vi "Drive Train.vi"(0 "C":dbl format="%#_13g", 1 "D":dbl format="%#_13g", 2 "X":dbl format="%#_13g", 3 "Y":dbl format="%#_13g", 4 "gyro":dbl, 6 "Mode Switch":bool, 7 "Positive 1":bool, 8 "Turning Switch":bool, 9 "Negative 1":bool=TRUE) -> (12 "gyro angle":dbl, 14 "A":dbl, 15 "B":dbl, 16 "R":dbl format="%#_13g")   [LabVIEW 2014]
panel:
  in  "alpha":dbl=1.0 step=0.1
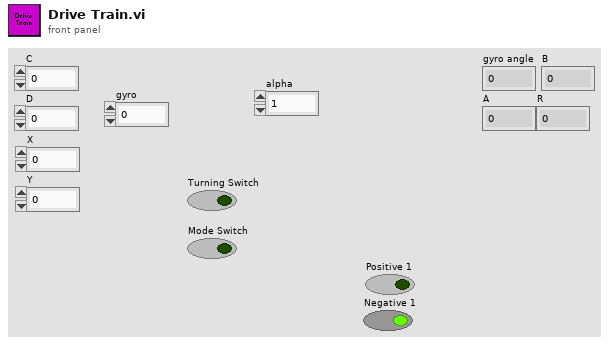
[diagram p1: front panel]
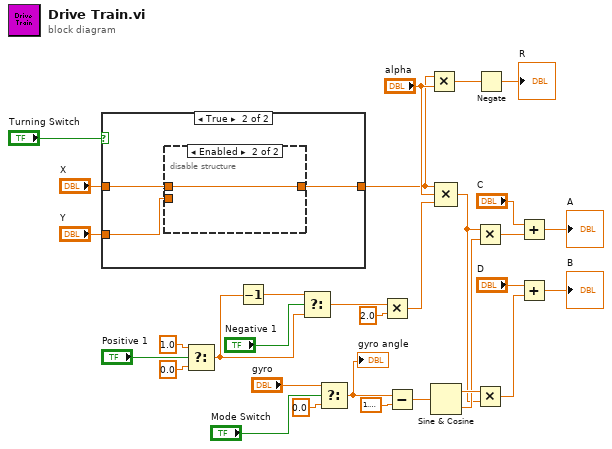
[diagram p0: block diagram]
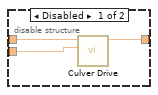
[diagram p3: hidden frame]
diagram:
  n1 = case shown="True" "Turning Switch" {
    tunnel: [w32 w33] -> w6
    tunnel: "X" -> [w32 w34]
    tunnel: "Y" -> [_ w35]
    frame False {
    }
    frame True {
      n2 = disable-structure shown="Enabled" {
        disable-tunnel: w35 -> [w38 _]
        disable-tunnel: w34 -> [w37 w39]
        disable-tunnel: [w36 w39] -> w33
        frame Disabled {
          n3 = call "Culver Drive.vi"("X"=w37, "Y"=w38) -> ("R"=w36:ext)  [unwired: 8 in]
        }
        frame Enabled {
        }
      }
    }
  }
  n4 = Select(t=1.0, s="Positive 1", f=0.0) -> (s? t:f=w15:dbl)
  n5 = Decrement(x=w15) -> (x-1=w14:dbl)
  n6 = Select(t=w14, s="Negative 1", f=w15) -> (s? t:f=w5:dbl)
  n7 = Select(t="gyro", s="Mode Switch", f=0.0 ("t")) -> (s? t:f=w23:dbl)
  "gyro angle" <- w23
  n8 = Multiply(x=w5, y=2.0) -> (x*y=w4:dbl)
  n9 = Subtract(x=w23, y=1.5707963267948966) -> (x-y=w13:dbl)
  n10 = Multiply(x=w6, y="alpha") -> (x*y=w2:dbl)
  n11 = Sine & Cosine(0:w13) -> (1:w11:dbl, 2:w8:dbl)
  n12 = Compound Arithmetic op=MULTIPLY(w6, "alpha", w4) -> (w7:dbl)
  n13 = Multiply(x=w7, y=w8) -> (x*y=w9:dbl)
  n14 = Multiply(x=w11, y=w7) -> (x*y=w10:dbl)
  n15 = Negate(x=w2) -> (-x=→"R":dbl)
  n16 = Add(x="C", y=w9) -> (x+y=→"A":dbl)
  n17 = Add(x="D", y=w10) -> (x+y=→"B":dbl)
